vi "efektivita.vi"() -> ()   [LabVIEW 2024]
uses:
  <vilib>/Analysis/baseanly.llb/Mean (DBL).vi
  <instrlib>/Zatez Kopper/Zatez Kopper.lvlib
  <instrlib>/EFmeter/EFmeter.lvlib
  <vilib>/Analysis/NI_AALBase.lvlib
panel:
  in  "Typ zateze":u16(ring) items=["Manualni", "BK 8542B", "KOPPER-zatez"]
  in  "EFmeter VISA":refnum<visa-resource-name>
  in  "Adresa souboru":path
  out "Aktualni zatez":dbl=2.5
  in  "Velikost kroku [A]":dbl
  in  "Start [A]":dbl
  in  "Prumerovani":bool
  in  "Vzorku na krokù":u16 max=100 step=1
  out "Zatezovaci charakteristika":cluster{"X":dbl[], "Y":dbl[]}[](graph)
  in  "Pocet kroku":i32
  in  "Clear":bool
  in  "Ulozit data":bool caption="Uložit data"
  in  "Start":bool
  in  "Zatez VISA":refnum<visa-resource-name>
  in  "stop":bool
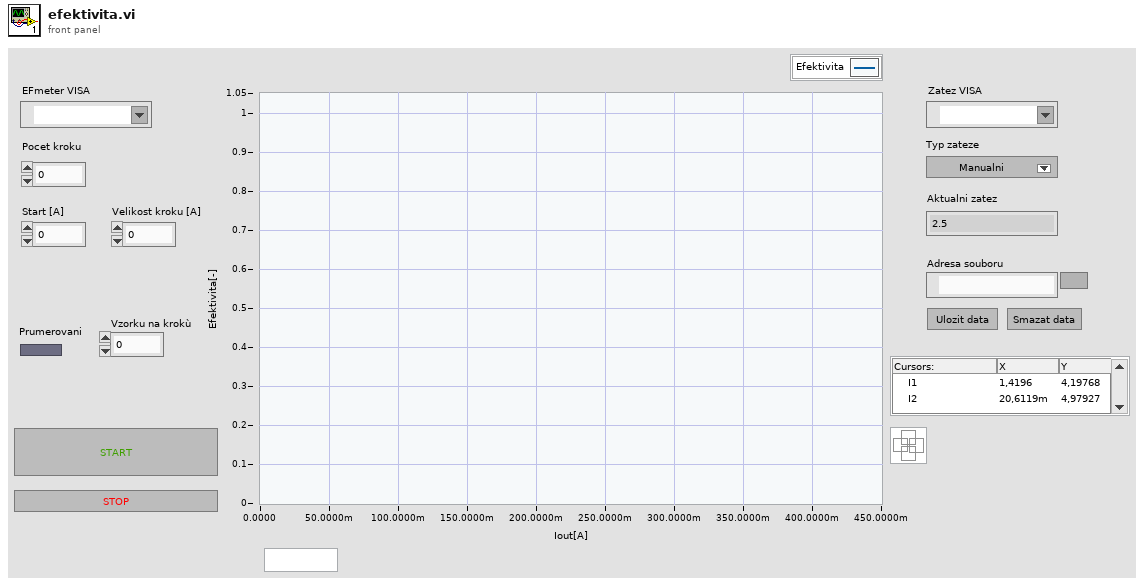
[diagram p1: front panel]
types:
  T1 = enum16{"open", "replace", "create", "open or create", "replace or create", "replace or create with confirmation"}
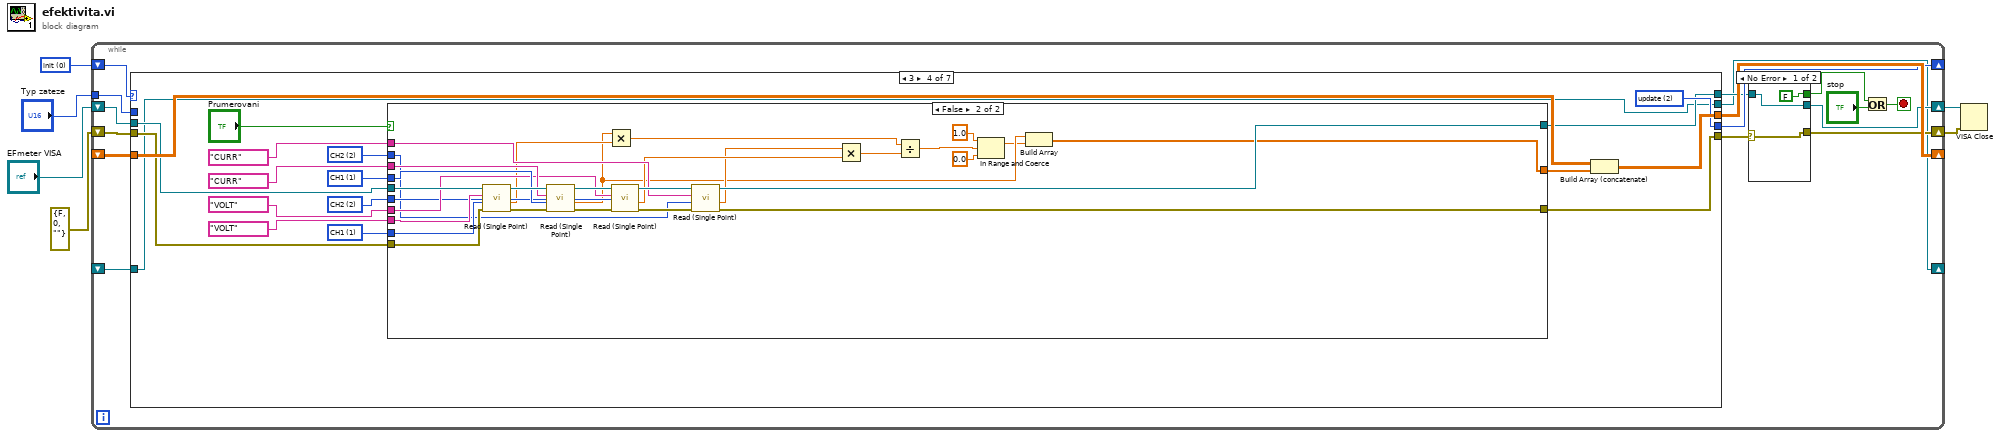
[diagram p0: block diagram]
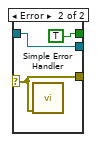
[diagram p2: hidden frame]
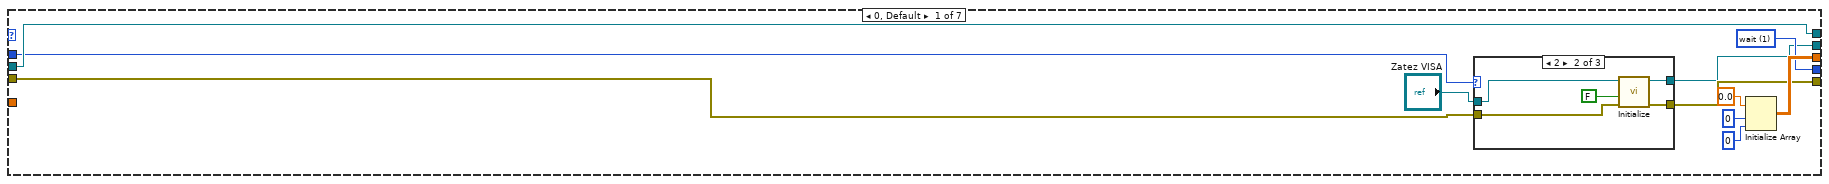
[diagram p3: hidden frame]
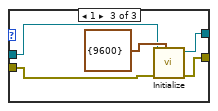
[diagram p5: hidden frame]
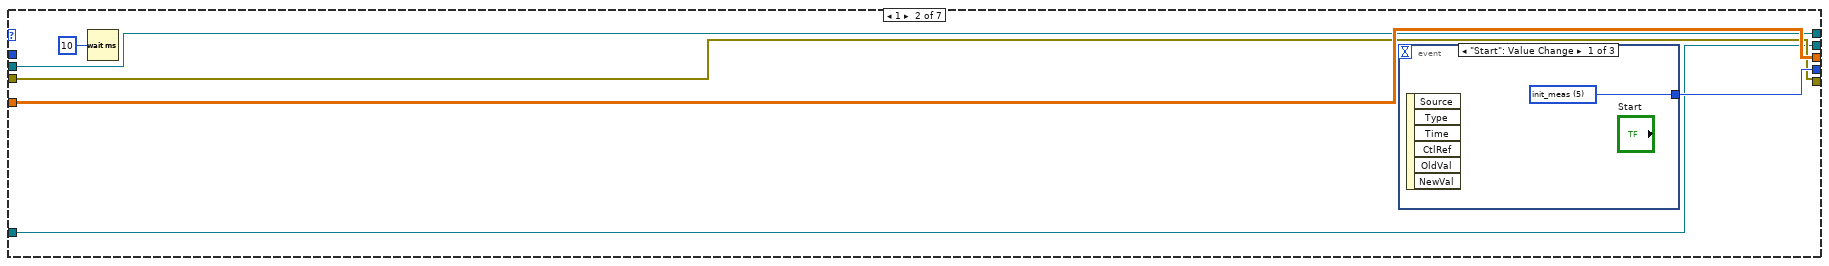
[diagram p6: hidden frame]
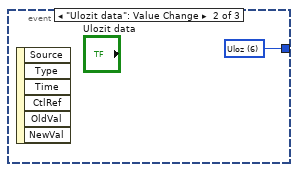
[diagram p7: hidden frame]
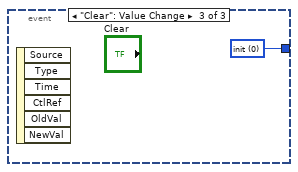
[diagram p8: hidden frame]
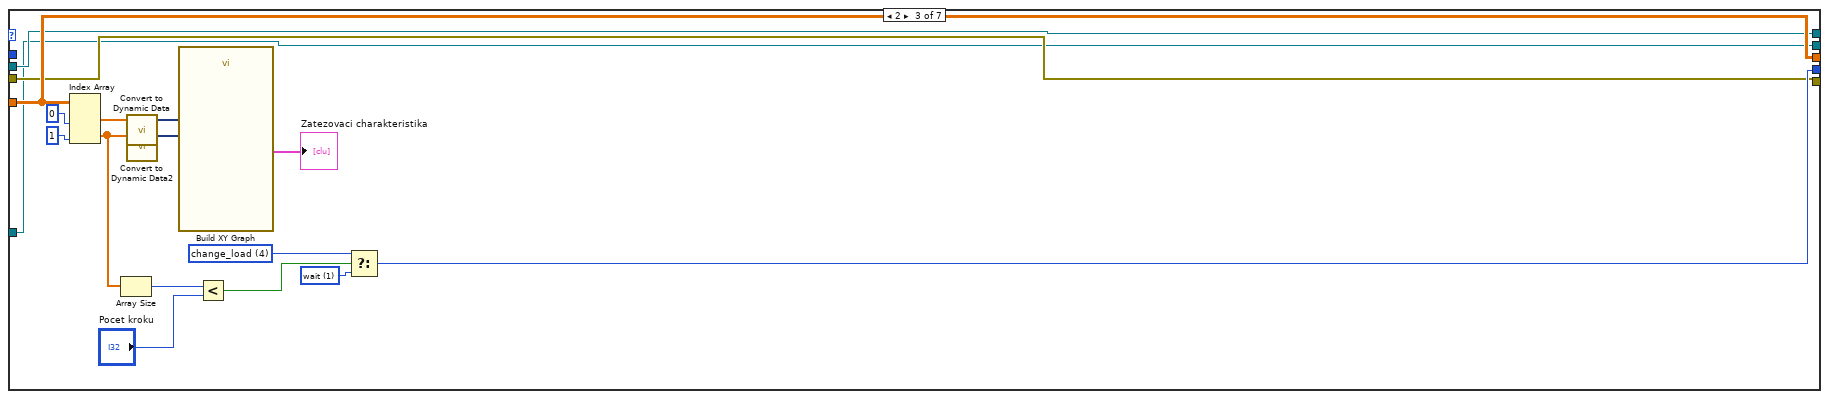
[diagram p9: hidden frame]
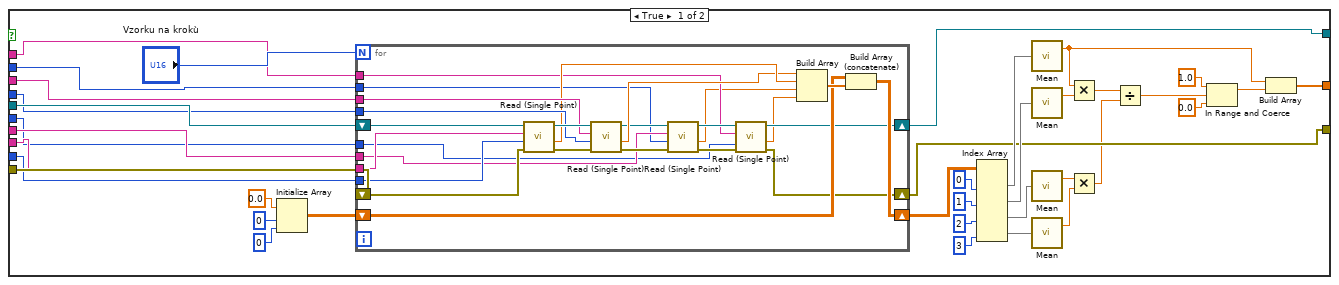
[diagram p10: hidden frame]
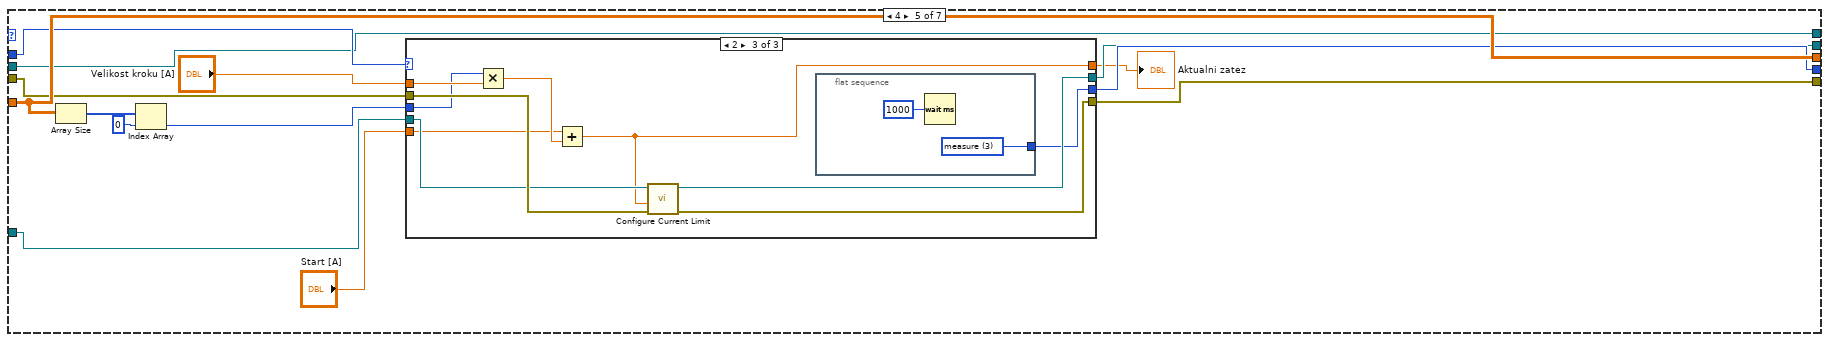
[diagram p11: hidden frame]
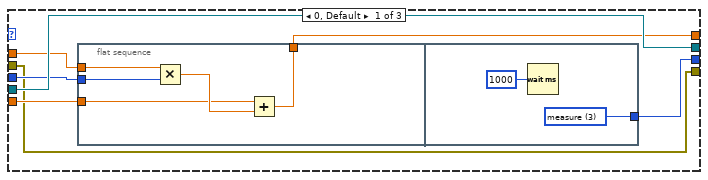
[diagram p12: hidden frame]
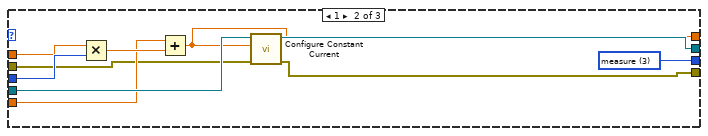
[diagram p13: hidden frame]
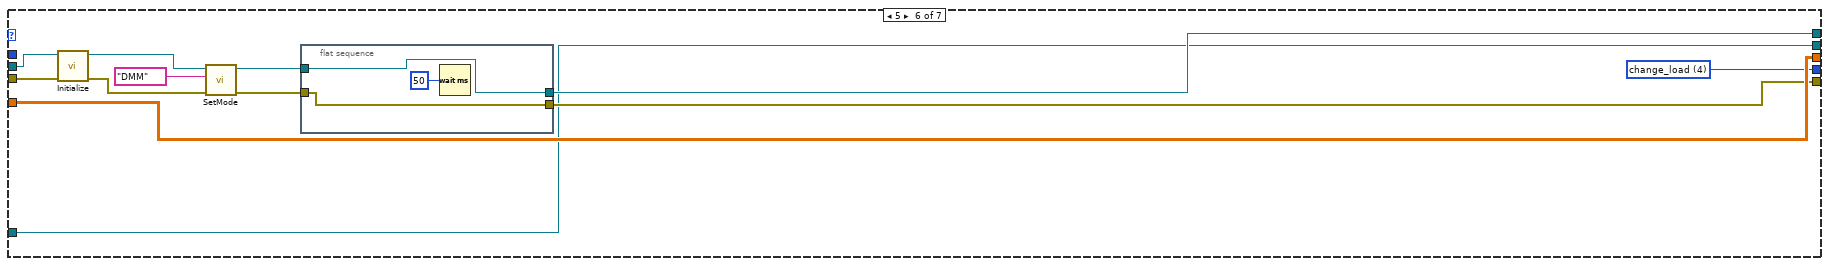
[diagram p14: hidden frame]
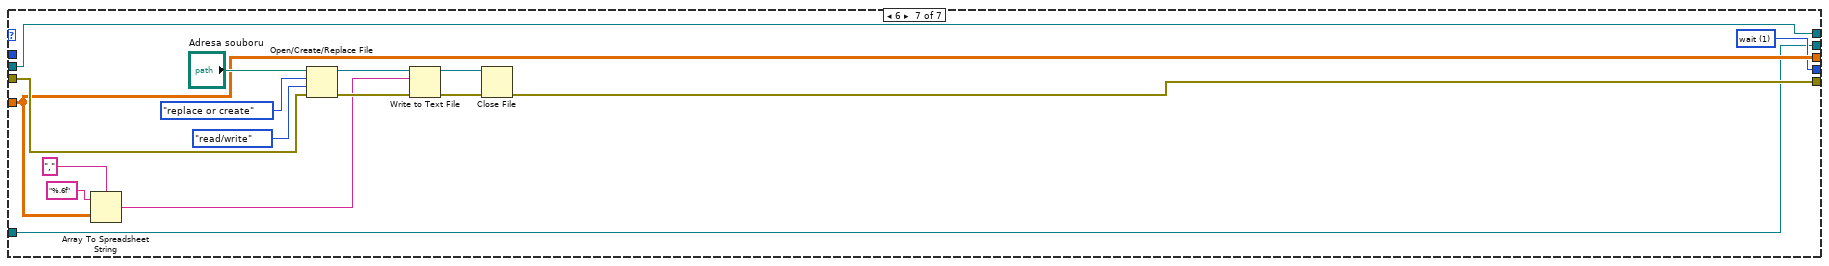
[diagram p15: hidden frame]
diagram:
  w6 = u16 0 items=["init", "wait", "update", "measure", "change_load", "init_meas", "Uloz", "clear"]
  n1 = while {
    shift-right: [w22] -> _
    shift-left: _ -> [w21]
    shift-right: [w17] -> _
    shift-left: w6 -> [w20]
    shift-right: [w14] -> w3
    shift-left: "EFmeter VISA" -> [w19]
    shift-right: [w13] -> w2
    shift-left: errorcluster {"status"=FALSE, "code"=0, "source"=""} ("error in (no error)") -> [w18]
    tunnel: "Typ zateze" -> [w9]
    shift-right: [w8] -> _
    shift-left: _ -> [w7]
    stop <- w11 stop-if-true
    n2 = case shown="3" w20 {
      tunnel: [w37 w56 w69 w94 w200 w248 w262] -> w22
      tunnel: w21 -> [_ w56 w69 w95 w200 w248 w262]
      tunnel: [w36 w57 w68 w92 w198 w247 w260] -> w17
      tunnel: [w33 w54 w62 w84 w188 w245 w256] -> w16
      tunnel: [w35 w55 w63 w85 w197 w246 w267] -> w15
      tunnel: w19 -> [w35 w55 w63 w91 w197 w242 w267]
      tunnel: w18 -> [w34 w54 w62 w90 w189 w243 w263]
      tunnel: w9 -> [w30 _ _ _ w199 _ _]
      tunnel: [w32 w52 w61 w82 w195 w244 w252] -> w8
      tunnel: w7 -> [_ w52 w61 w82 w196 w244 w252]
      frame 0, Default {
        w36 = u16 1 items=["init", "wait", "update", "measure"]
        n3 = case shown="2" w30 {
          tunnel: w34 -> [w41 w45 w50]
          tunnel: [w41 w44 w49] -> w33
          tunnel: [w40 w43 w48] -> w32
          tunnel: "Zatez VISA" -> [w40 w46 w47]
          frame 0, Default {
          }
          frame 2 {
            n4 = call <instrlib>:"Initialize.vi"("error in (no error)"=w45, "Reset (True)"=FALSE, "VISA resource name"=w46) -> ("error out"=w44:errorcluster, "VISA resource name out"=w43:refnum<visa-resource-name>)  [unwired: 7 in]
          }
          frame 1 {
            n5 = call <instrlib>:"Initialize.vi"("Serial Configuration"=cluster{"Baud Rate":u32} {"Baud Rate"=9600}, "error in (no error)"=w50, "VISA resource name"=w47) -> ("error out"=w49:errorcluster, "VISA resource name out"=w48:refnum<visa-resource-name>)  [unwired: 7 in]
          }
        }
        n6 = Initialize Array(0.0 ("element"), 0 ("dimension size"), 0 ("dimension size")) -> (w37:dbl[][])
      }
      frame 1 {
        n7 = Wait (ms)(milliseconds to wait=u32 10) -> ()  [unwired: 1 out]
        n8 = event shown="[0] \"Start\": Value Change" {
          selector: _ -> [_ _ _]
          dyn-events: _ -> [_ _ _]
          timeout: _ -> [_ _ _]
          tunnel: [w58 w59 w60] -> w57
          event "Start": Value Change {
            w58 = u16 5 items=["init", "wait", "update", "measure", "change_load", "init_meas"]
            n9 = event-data() -> ()  [unwired: 1 in, 6 out]
          }
          event "Ulozit data": Value Change {
            w59 = u16 6 items=["init", "wait", "update", "measure", "change_load", "init_meas", "Uloz"]
            n10 = event-data() -> ()  [unwired: 1 in, 6 out]
          }
          event "Clear": Value Change {
            w60 = u16 0 items=["init", "wait", "update", "measure", "change_load", "init_meas", "Uloz", "clear"]
            n11 = event-data() -> ()  [unwired: 1 in, 6 out]
          }
        }
      }
      frame 2 {
        w64 = u16 4 items=["init", "wait", "update", "measure", "change_load", "init_meas"]
        w70 = u16 1 items=["init", "wait", "update", "measure"]
        n12 = Index Array(array=w69, index (col) #1=0 ("index (row)"), index (col) #2=1 ("index (row)")) -> (element #1=w77:dbl[], element #2=w72:dbl[])  [unwired: 2 in]
        n13 = Array Size(array=w72) -> (size(s)=w74:i32)
        n14 = call "Convert to Dynamic Data"("Array"=w77) -> ("Dynamic Data Type"=w76:dynamicdata)  [unwired: 3 in]
        n15 = call "Convert to Dynamic Data2"("Array"=w72) -> ("Dynamic Data Type"=w75:dynamicdata)  [unwired: 3 in]
        n16 = call "Build XY Graph"("Y Input"=w75, "X Input"=w76) -> ("XY Graph"=→"Zatezovaci charakteristika":cluster{"X":dbl[], "Y":dbl[]}[])  [unwired: 8 in, 1 out]
        n17 = Less?(x=w74, y="Pocet kroku") -> (x < y?=w73:bool)
        n18 = Select(t=w64, s=w73, f=w70) -> (s? t:f=w68:u16)
      }
      frame 3 {
        w78 = u16 2 items=["CH2"=2, "CH1"=1] ("Ring")
        w79 = u16 2 items=["CH2"=2, "CH1"=1] ("Ring")
        w86 = u16 1 items=["CH2"=2, "CH1"=1] ("Ring")
        w89 = u16 1 items=["CH2"=2, "CH1"=1] ("Ring")
        w92 = u16 2 items=["init", "wait", "update", "measure"]
        n19 = case shown="False" "Prumerovani" {
          tunnel: [w100 w162] -> w93
          tunnel: w91 -> [w127 w186]
          tunnel: w90 -> [w126 w185]
          tunnel: w89 -> [w125 w184]
          tunnel: "VOLT" ("Combo Box") -> [w124 w183]
          tunnel: "CURR" ("Combo Box") -> [w123 w180]
          tunnel: w86 -> [w122 w179]
          tunnel: [w116 w174] -> w85
          tunnel: [w115 w173] -> w84
          tunnel: "VOLT" ("Combo Box") -> [w113 w172]
          tunnel: "CURR" ("Combo Box") -> [w112 w170]
          tunnel: w79 -> [w111 w169]
          tunnel: w78 -> [w110 w171]
          frame True {
            n20 = Initialize Array(0.0 ("element"), 0 ("dimension size"), 0 ("dimension size")) -> (w128:dbl[][])
            n21 = for {
              N: "Vzorku na krokù" -> [_]
              shift-right: [w139] -> w116
              shift-left: w127 -> [w153]
              shift-right: [w140] -> w115
              shift-left: w126 -> [w152]
              tunnel: w125 -> [w151]
              tunnel: w124 -> [w150]
              tunnel: w123 -> [w149]
              tunnel: w122 -> [w148]
              shift-right: [w147] -> w121
              shift-left: w128 -> [w154]
              tunnel: w113 -> [w138]
              tunnel: w112 -> [w137]
              tunnel: w111 -> [w136]
              tunnel: w110 -> [w135]
              n22 = call <instrlib>:"Read (Single Point).vi"("error in (no error)"=w152, "Ring"=w151, "Combo Box"=w150, "VISA resource name"=w153) -> ("error out"=w156:errorcluster, "Measurement"=w146:dbl, "VISA resource name out"=w157:refnum<visa-resource-name>)  [unwired: 5 in]
              n23 = call <instrlib>:"Read (Single Point).vi"("error in (no error)"=w156, "Ring"=w148, "Combo Box"=w149, "VISA resource name"=w157) -> ("error out"=w144:errorcluster, "Measurement"=w145:dbl, "VISA resource name out"=w143:refnum<visa-resource-name>)  [unwired: 5 in]
              n24 = call <instrlib>:"Read (Single Point).vi"("error in (no error)"=w144, "Ring"=w136, "Combo Box"=w138, "VISA resource name"=w143) -> ("error out"=w141:errorcluster, "Measurement"=w134:dbl, "VISA resource name out"=w142:refnum<visa-resource-name>)  [unwired: 5 in]
              n25 = call <instrlib>:"Read (Single Point).vi"("error in (no error)"=w141, "Ring"=w135, "Combo Box"=w137, "VISA resource name"=w142) -> ("error out"=w140:errorcluster, "Measurement"=w133:dbl, "VISA resource name out"=w139:refnum<visa-resource-name>)  [unwired: 5 in]
              n26 = Build Array(w145, w146, w134, w133) -> (w155:dbl[])
              n27 = Build Array (concatenate)(w154, w155) -> (w147:dbl[][])
            }
            n28 = Index Array(array=w121, index (col) #1=0 ("disabled index (col)"), index (col) #2=1 ("index (col)"), index (col) #3=2 ("index (col)"), index (col) #4=3 ("index (col)")) -> (element #1=w120:dbl[], element #2=w119:dbl[], element #3=w107:dbl[], element #4=w106:dbl[])  [unwired: 4 in]
            n29 = call-poly <vilib>:"Mean.vi"("X"=w120) -> ("mean"=w101:dbl)  [unwired: 1 out]
            n30 = call-poly <vilib>:"Mean.vi"("X"=w119) -> ("mean"=w114:dbl)  [unwired: 1 out]
            n31 = call-poly <vilib>:"Mean.vi"("X"=w107) -> ("mean"=w104:dbl)  [unwired: 1 out]
            n32 = call-poly <vilib>:"Mean.vi"("X"=w106) -> ("mean"=w105:dbl)  [unwired: 1 out]
            n33 = Multiply(x=w101, y=w114) -> (x*y=w102:dbl)
            n34 = Multiply(x=w104, y=w105) -> (x*y=w103:dbl)
            n35 = Divide(x=w102, y=w103) -> (x/y=w98:dbl)
            n36 = In Range and Coerce(upper limit=1.0, x=w98, lower limit=0.0) -> (coerced(x)=w99:dbl)  [unwired: 1 out]
            n37 = Build Array(w101, w99) -> (w100:dbl[])
          }
          frame False {
            n38 = call <instrlib>:"Read (Single Point).vi"("error in (no error)"=w185, "Ring"=w184, "Combo Box"=w183, "VISA resource name"=w186) -> ("error out"=w182:errorcluster, "Measurement"=w168:dbl, "VISA resource name out"=w181:refnum<visa-resource-name>)  [unwired: 5 in]
            n39 = call <instrlib>:"Read (Single Point).vi"("error in (no error)"=w182, "Ring"=w179, "Combo Box"=w180, "VISA resource name"=w181) -> ("error out"=w177:errorcluster, "Measurement"=w163:dbl, "VISA resource name out"=w178:refnum<visa-resource-name>)  [unwired: 5 in]
            n40 = Multiply(x=w163, y=w168) -> (x*y=w165:dbl)
            n41 = call <instrlib>:"Read (Single Point).vi"("error in (no error)"=w177, "Ring"=w171, "Combo Box"=w172, "VISA resource name"=w178) -> ("error out"=w175:errorcluster, "Measurement"=w167:dbl, "VISA resource name out"=w176:refnum<visa-resource-name>)  [unwired: 5 in]
            n42 = call <instrlib>:"Read (Single Point).vi"("error in (no error)"=w175, "Ring"=w169, "Combo Box"=w170, "VISA resource name"=w176) -> ("error out"=w173:errorcluster, "Measurement"=w166:dbl, "VISA resource name out"=w174:refnum<visa-resource-name>)  [unwired: 5 in]
            n43 = Multiply(x=w166, y=w167) -> (x*y=w164:dbl)
            n44 = Divide(x=w165, y=w164) -> (x/y=w161:dbl)
            n45 = In Range and Coerce(upper limit=1.0, x=w161, lower limit=0.0) -> (coerced(x)=w160:dbl)  [unwired: 1 out]
            n46 = Build Array(w163, w160) -> (w162:dbl[])
          }
        }
        n47 = Build Array (concatenate)(w95, w93) -> (w94:dbl[][])
      }
      frame 4 {
        n48 = Array Size(array=w200) -> (size(s)=w190:i32[])
        n49 = Index Array(array=w190, index=0) -> (element=w192:i32)
        n50 = case shown="2" w199 {
          tunnel: [w207 w224 w226] -> w198
          tunnel: w196 -> [w206 w223 w231]
          tunnel: [w206 w222 w234] -> w195
          tunnel: "Velikost kroku [A]" -> [w205 w220 w229]
          tunnel: "Start [A]" -> [w204 w218 w228]
          tunnel: w192 -> [w203 w221 w227]
          tunnel: w189 -> [w202 w217 w232]
          tunnel: [w202 w216 w233] -> w188
          tunnel: [w201 w215 w225] -> w187
          frame 0, Default {
            n51 = flat-sequence {
              tunnel: w205 -> [w211]
              tunnel: w204 -> [w210]
              tunnel: w203 -> [w209]
              tunnel: [w208] -> w201
              tunnel: [w214] -> w207
              frame #0 {
                n52 = Multiply(x=w211, y=w209) -> (x*y=w212:dbl)
                n53 = Add(x=w210, y=w212) -> (x+y=w208:dbl)
              }
              frame #1 {
                w214 = u16 3 items=["init", "wait", "update", "measure", "change_load", "init_meas"]
                n54 = Wait (ms)(milliseconds to wait=u32 1000) -> ()  [unwired: 1 out]
              }
            }
          }
          frame 1 {
            w224 = u16 3 items=["init", "wait", "update", "measure", "change_load", "init_meas"]
            n55 = Multiply(x=w220, y=w221) -> (x*y=w219:dbl)
            n56 = Add(x=w218, y=w219) -> (x+y=w215:dbl)
            n57 = call "Configure Constant Current.vi"("error in (no error)"=w217, "CC Current (0)"=w215, "VISA resource name"=w223) -> ("error out"=w216:errorcluster, "VISA resource name out"=w222:refnum<visa-resource-name>)  [unwired: 7 in]
          }
          frame 2 {
            n58 = Multiply(x=w227, y=w229) -> (x*y=w230:dbl)
            n59 = Add(x=w228, y=w230) -> (x+y=w225:dbl)
            n60 = call <instrlib>:"Configure Current Limit.vi"("error in (no error)"=w232, "Current Limit (0.0 A)"=w225, "VISA resource name"=w231) -> ("error out"=w233:errorcluster, "VISA resource name out"=w234:refnum<visa-resource-name>)  [unwired: 7 in]
            n61 = flat-sequence {
              tunnel: [w236] -> w226
              frame #0 {
                w236 = u16 3 items=["init", "wait", "update", "measure", "change_load", "init_meas"]
                n62 = Wait (ms)(milliseconds to wait=u32 1000) -> ()  [unwired: 1 out]
              }
            }
          }
        }
        "Aktualni zatez" <- w187
      }
      frame 5 {
        w247 = u16 4 items=["init", "wait", "update", "measure", "change_load", "init_meas"]
        n63 = call <instrlib>:"Initialize.vi"("error in (no error)"=w243, "VISA resource name"=w242) -> ("error out"=w239:errorcluster, "VISA resource name out"=w240:refnum<visa-resource-name>)  [unwired: 8 in]
        n64 = call <instrlib>:"SetMode.vi"("error in (no error)"=w239, "Combo Box"="DMM", "VISA resource name"=w240) -> ("error out"=w238:errorcluster, "VISA resource name out"=w237:refnum<visa-resource-name>)  [unwired: 7 in]
        n65 = flat-sequence {
          tunnel: [w250] -> w246
          tunnel: w237 -> [w250]
          tunnel: w238 -> [w249]
          tunnel: [w249] -> w245
          frame #0 {
            n66 = Wait (ms)(milliseconds to wait=u32 50) -> ()  [unwired: 1 out]
          }
        }
      }
      frame 6 {
        w260 = u16 1 items=["init", "wait", "update", "measure", "change_load", "init_meas"]
        n67 = Array To Spreadsheet String(delimiter (Tab)=",", array=w262, 3:"%.6f" ("format string")) -> (spreadsheet string=w253:string)
        n68 = Open/Create/Replace File(file path (use dialog)="Adresa souboru", error in=w263, operation (0:open)=T1."replace or create", access (0:read/write)=enum16{"read/write", "read-only", "write-only"}."read/write") -> (refnum out=w255:refnum<file>, error out=w258:errorcluster)  [unwired: 2 in, 1 out]
        n69 = Write to Text File(file (use dialog)=w255, text=w253, error in=w258) -> (refnum out=w254:refnum<file>, error out=w257:errorcluster)  [unwired: 1 in, 1 out]
        n70 = Close File(refnum=w254, error in=w257) -> (error out=w256:errorcluster)  [unwired: 1 out]
      }
    }
    n71 = case shown="No Error" w16 {
      selector: w16 -> [w24 w26]
      tunnel: w15 -> [w25 w28]
      tunnel: [w25 w28] -> w14
      tunnel: [w24 w26] -> w13
      tunnel: [FALSE TRUE] -> w10
      frame No Error {
      }
      frame Error {
        n72 = call <vilib>:"Simple Error Handler.vi"("error in (no error)"=w26) -> ()  [unwired: 4 in, 5 out]
      }
    }
    n73 = Or(x=w10, y="stop") -> (x .or. y?=w11:bool)
  }
  n74 = VISA Close(VISA resource name=w3, error in (no error)=w2) -> ()  [unwired: 1 out]
